vi "Get Report File Path.vi"(0 "Path":path) -> (2 "Report File":path)   [LabVIEW 2019, in "Caraya Library.lvlib" / "Run Tests Step.lvclass"]
doc: "Returns the path to a report file in the user's temp folder."
uses:
  Run Tests Step.lvclass
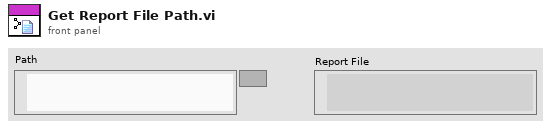
[diagram p1: front panel]
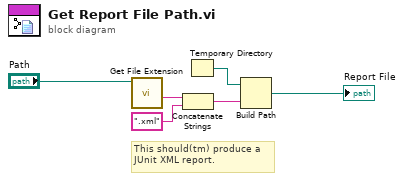
[diagram p0: block diagram]
diagram:
  # "This should(tm) produce a\nJUnit XML report."
  n1 = call <vilib>:"Get File Extension.vi"("file"="Path") -> ("filename without extension"=w3:string)  [unwired: 6 in, 4 out]
  n2 = Concatenate Strings(w3, ".xml" ("Temporary File Extension (tmp)")) -> (w4:string)
  n3 = Temporary Directory() -> (w6:path)
  n4 = Build Path(base path=w6, name or relative path=w4) -> (appended path=→"Report File":path)
